vi "Intake Global.vi"() -> ()   [LabVIEW 2013]
uses:
  <vilib>/Rock Robotics/WPI/Solenoid/WPI_SolenoidValue.ctl
panel:
  in  "Intake Info":T2
  # "True = Out\nFalse = In"
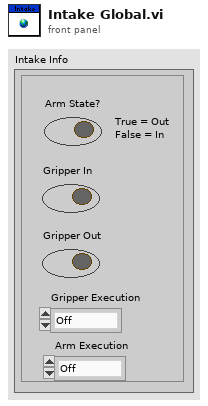
[diagram p1: front panel]
types:
  T1 = typedef "WPI_SolenoidValue.ctl" = enum16{"Off", "On", "Forward", "Reverse"}
  T2 = cluster{"Arm State?":bool, "Gripper In":bool, "Gripper Out":bool, "Gripper Execution ":T1, "Arm Execution ":T1}
diagram:
